vi "InitiateGenerationV01.vi"(8 "error in (no error)":errorcluster, 11 "ClassIn":refnum<class "Keysight335XX.lvclass">) -> (0 "error out":errorcluster, 3 "ClassOut":refnum<class "Keysight335XX.lvclass">)   [LabVIEW 2014, in "FGenPlugins.lvlib" / "Keysight335XX.lvclass"]
uses:
  Keysight335XX.lvclass
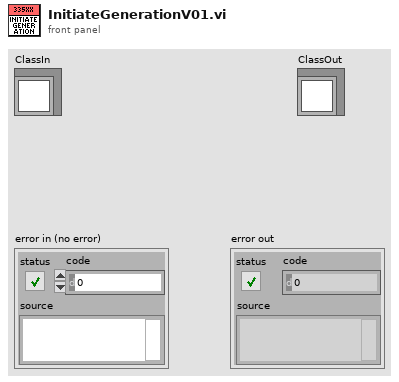
[diagram p1: front panel]
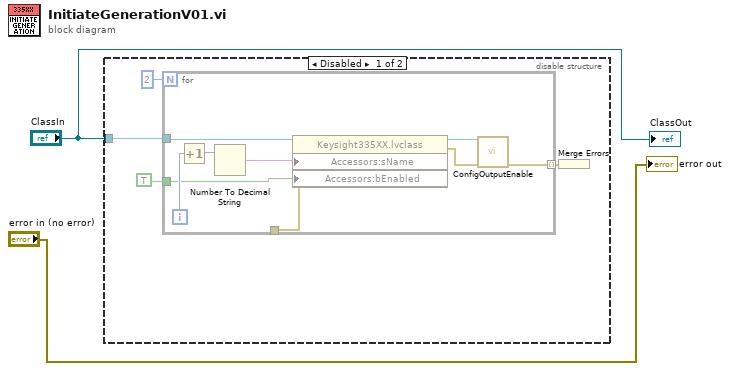
[diagram p0: block diagram]
diagram:
  n1 = disable-structure shown="Disabled" {
    disable-tunnel: "ClassIn" -> [w7 _]
    frame Disabled {
      n2 = for {
        N: 2 -> [_]
        tunnel: w7 -> [w15]
        tunnel: TRUE -> [w12]
        tunnel: [w11] -> w3
        tunnel: [w8] -> w6 mode=indexing
        i -> [w14]
        n3 = Increment(x=w14) -> (x+1=w13:i32)
        n4 = Number To Decimal String(number=w13) -> (decimal integer string=w16:string)  [unwired: 1 in]
        n5 = property class="Keysight335XX.lvclass"(reference=w15, error in=w11, "Accessors:sName"=w16, "Accessors:bEnabled"=w12) -> (reference out=w9:refnum<class "Keysight335XX.lvclass">, error out=w10:errorcluster)
        n6 = call-dynamic "ConfigOutputEnable.vi"("error in (no error)"=w10, "ClassIn"=w9) -> ("error out"=w8:errorcluster)  [unwired: 8 in, 1 out]
      }
      n7 = Merge Errors(w6) -> ()  [unwired: 1 out]
    }
    frame Enabled {
    }
  }
  "error out" <- "error in (no error)"
  "ClassOut" <- "ClassIn"
